vi "Special Test, Record Results.vi"(7 "step name":string="Pulse Attribute Results", 8 "error in":errorcluster, 10 "results":T1[](array[typedef])=[{"Label"="Stim Amp (mA)", "Value"=nan}, {"Label"="Stim Pulse Width (us)", "Value"=nan}, {"Label"="Interphase Delay (us)", "Value"=nan}, {"Label"="Recvy Amp (mA)", "Value"=nan}, {"Label"="Recvy Pulse Width (us)", "Value"=nan}, {"Label"="Frequency (Hz)", "Value"=nan}, {"Label"="Period Jitter (us rms)", "Value"=nan}] {"Value" format="%#.3f"}, 11 "Sequence Context":refnum<k7>) -> (0 "error out":errorcluster, 3 "Sequence Context dup":refnum<k7>)   [LabVIEW 2010]
doc: "This function transfers a single Compare Data Test (CDT) record to the current TestStand sequence step."
uses:
  Generic/Waveform Attribute/Waveform Attribute Cluster.ctl
panel:
  in  "Acceptance Criteria":string[][](table)=[["TRS1763", "Stimulus Phase Amplitude", "", "-5.170", "-4.830", "mA", "GELE", "%.3f", "%.3f", "TC1"], ["TRS1762", "Stimulus Phase Pulse Width", "", "92.0", "108.0", "us", "GELE", "%.2f", "%.2f", "TC1"], ["TRS1761", "Active Interphase Delay", "", "13.0", "27.0", "us", "GELE", "%.1f", "%.1f", "TC1"], ["TRS1760", "Active Recovery Phase Amplitude", "", "4.830", "5.170", "mA", "GELE", "%.3f", "%.3f", "TC1"], ["TRS1759", "Active Recovery Phase Pulse Width", "", "95.0", "105.0", "us", "GELE", "%.1f", "%.1f", "TC1"], ["TRS1758", "Frequency", "", "965.0", "1035.0", "Hz", "GELE", "%.1f", "%.1f", "TC1"], ["TRS1757", "Pulse Period Jitter (RMS)", "", "-2.500", "2.500", "us", "GELE", "%.1f", "%.1f", "TC1"]] caption="Table 1"
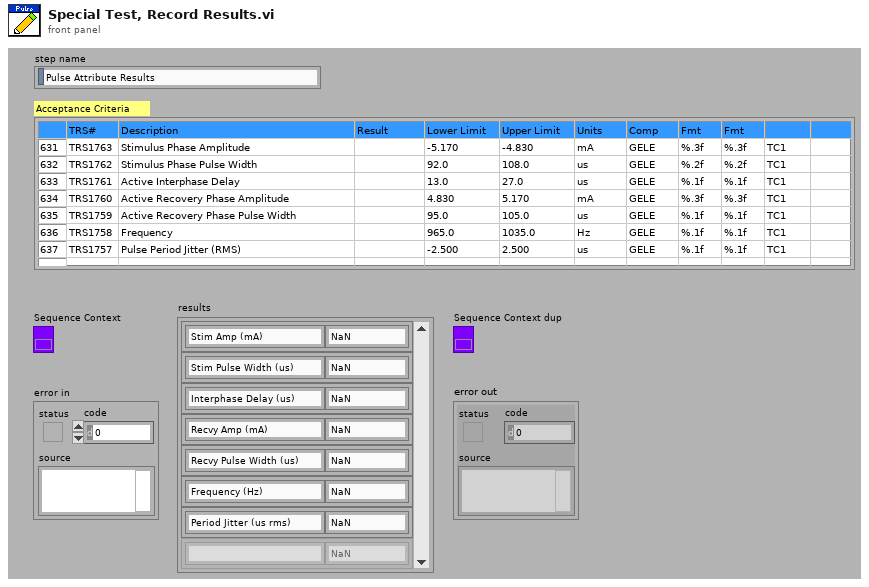
[diagram p1: front panel]
types:
  T1 = typedef "Waveform Attribute Cluster.ctl" = cluster{"Label":string, "Value":dbl}
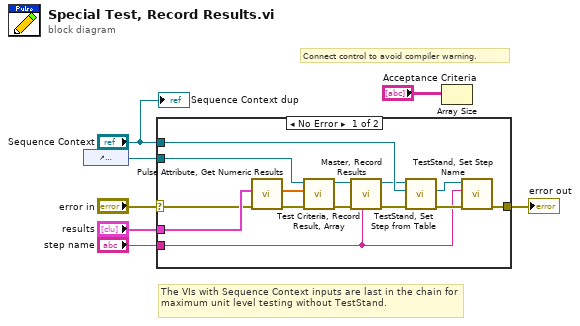
[diagram p0: block diagram]
diagram:
  # "The VIs with Sequence Context inputs are last in the chain for maximum unit level testing without TestStand."
  # "Connect control to avoid compiler warning."
  n1 = control-ref of="Acceptance Criteria"() -> (w3:refnum<vi>)
  n2 = case shown="No Error" "error in" {
    selector: "error in" -> [w9 w22]
    tunnel: [w17 w22] -> w7
    tunnel: "Sequence Context" -> [w16 _]
    tunnel: w3 -> [w8 _]
    tunnel: "results" -> [w20 _]
    tunnel: "step name" -> [w10 _]
    frame No Error {
      n3 = call "Pulse Attribute, Get Numeric Results.vi"("error in"=w9, "results"=w20) -> ("error out"=w21:errorcluster, "numeric values"=w19:dbl[])  [unwired: 4 in]
      n4 = call "Test Criteria, Record Result, Array.vi"("error in"=w21, "Results"=w19, "Tbl Refnum"=w8) -> ("error out"=w14:errorcluster, "Tbl Refnum out"=w12:refnum<vi>)  [unwired: 6 in, 1 out]
      n5 = call "Master, Record Results.vi"("step name"=w10, "error in"=w14, "Tbl Refnum"=w12) -> ("error out"=w13:errorcluster, "Tbl Refnum dup"=w11:refnum<vi>)  [unwired: 7 in]
      n6 = call "TestStand, Set Step from Table.vi"("error in"=w13, "Sequence Context"=w16, "Tbl Refnum"=w11) -> ("error out"=w18:errorcluster, "Sequence Context Out"=w15:refnum<k7>)  [unwired: 6 in, 1 out]
      n7 = call "TestStand, Set Step Name.vi"("error in"=w18, "Step Name"=w10, "Sequence Context"=w15) -> ("error out"=w17:errorcluster)  [unwired: 7 in, 1 out]
    }
    frame Error {
    }
  }
  "error out" <- w7
  n8 = Array Size(array="Acceptance Criteria") -> ()  [unwired: 1 out]
  "Sequence Context dup" <- "Sequence Context"
